vi "Disable All.vi"(8 "error in":errorcluster) -> (0 "error out":errorcluster)   [LabVIEW 2018, in "GLog.lvlib" / "Registry.lvlib"]
uses:
  Registry.lvlib
  Registry Actions.ctl
panel:
  # "Connector Pane"
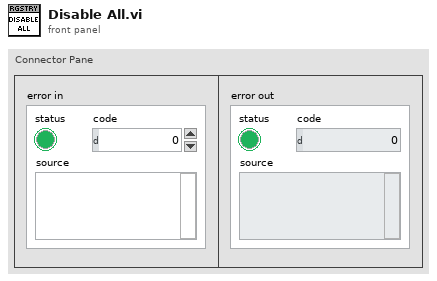
[diagram p1: front panel]
types:
  T1 = typedef "GLog.lvlib/Registry.lvlib/Registry Actions.ctl" = enum16{"Register", "Log", "Enable", "Enable All", "Disable", "Disable All", "List", "Unregister", "Unregister All", "Shutdown"}
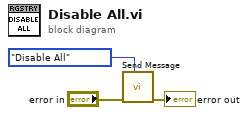
[diagram p0: block diagram]
diagram:
  n1 = call "Send Message.vi"("action"=Registry_Actions."Disable All", "error in (no error)"="error in") -> ("error out"=→"error out":errorcluster)  [unwired: 9 in]
